vi "PH_ImageCoG_Plotter.PC Set Beam Analysis.vi"(0 "i ref in":refnum<vi>, 2 "On / Off":bool, 5 "error in (no error)":errorcluster) -> (14 "i ref out":refnum<vi>, 19 "error out":errorcluster)   [LabVIEW 2014, in "PH_ImageCoG_Plotter.lvlib"]
doc: "This VI writes beam analysis settings to own attributes and sets the GUI elements."
uses:
  PH_ImageCoG_Plotter.lvlib
  PH_Common/PH_Common.lvlib
  CSCore/BaseProcess/BaseProcess.lvlib
  PH_Img_BaseClass/PH_Img_BaseClass.lvlib
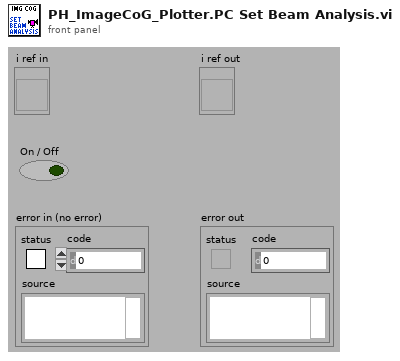
[diagram p1: front panel]
types:
  T1 = typedef "PH_ImageCoG_Plotter.lvlib/PH_ImageCoG_Plotter.i attribute.ctl" = cluster{"GUI Refs":cluster{"Delete":refnum<vi>, "Calibration status":refnum<vi>, "BI subtracted":refnum<vi>, "calc Beam Anal":refnum<vi>, "CoG - x":refnum<vi>, "CoG - y":refnum<vi>, "Type":refnum<vi>, "Center":refnum<vi>, "exp - X":refnum<vi>, "exp - Y":refnum<vi>, "Delta - X":refnum<vi>, "Delta - Y":refnum<vi>, "Available Cams":refnum<vi>, "CoG X":refnum<vi>, "CoG Y":refnum<vi>, "Delta X":refnum<vi>, "Delta Y":refnum<vi>, "Export Data":refnum<vi>, "Calibration data":refnum<vi>}, "Calibration":cluster{"Status":T2, "Calibration data":T3, "Calibration Data File":path}, "Beam Analysis":cluster{"on":bool, "exp - X":i32, "exp - Y":i32, "Type":bool, "Data":cluster{"current time":timestamp, "CoG-x":dbl, "CoG-y":dbl, "Delta-x":dbl, "Delta-y":dbl}[], "Datasets strored":i32, "Dataarray Size":i32}, "Cam instances":string[], "DIM Service Events":T4[], "Images":cluster{"Background":T7, "OP":T7, "GUI":T7}}
  T2 = typedef "PH_StatusHandler.lvlib/PH_StatusHandler.Status.ctl" = i16
  T3 = typedef "PH_ImageCalibrator.lvlib/PH_ImageCalibrator.Calibration Data.ctl" = cluster{"Date":string, "Time":string, "Cam Settings":cluster{"Cam ID":string, "Gain":dbl, "Brightness":dbl, "Shutter":dbl, "Cam Error":bool, "Mode":i32}, "Background Image":cluster{"Image":dbl[][], "Image Error":bool}, "Linear Calibration":cluster{"Calibration Factor":dbl, "not mm or mrad":bool}, "Energy Calibration":cluster{"Calibration Factor":dbl, "no mJ":bool}}
  T4 = typedef "BaseProcess.lvlib/BaseProcess.event definition.ctl" = cluster{"CAEEvtDef":T5, "Data Descriptor":T6}
  T5 = typedef "CAEObj.lvlib/CAEObj.event definition.ctl" = cluster{"URL":string, "enable":bool, "ignoreResID":bool}
  T6 = typedef "BaseProcess.lvlib/BaseProcess.descriptor string definition.ctl" = string
  T7 = typedef "IMAQ Image.ctl" = refnum<image>
  T8 = typedef "PH_Img_BaseClass.lvlib/PH_Img_BaseClass.i attribute.ctl" = cluster{"GUI Refs":T9, "Timeout Image [ms]":i32, "Default Periodic Period [ms]":i32, "Camera":cluster{"Instancename":string, "Notifier":refnum<notifier>}, "Palette":T10, "Cam Settings":cluster{"Cam ID":string, "Gain":dbl, "Brightness":dbl, "Shutter":dbl, "Cam Info Failure":bool, "Mode":i32}}
  T9 = typedef "PH_Img_BaseClass.lvlib/PH_Img_BaseClass.GUI Refs.ctl" = cluster{"Timeout":refnum<vi>, "Image":refnum<vi>, "Palette":refnum<vi>, "Timeout Set":refnum<vi>}
  T10 = typedef "PH_Img_BaseClass.lvlib/PH_Img_BaseClass.Palette.ctl" = i32
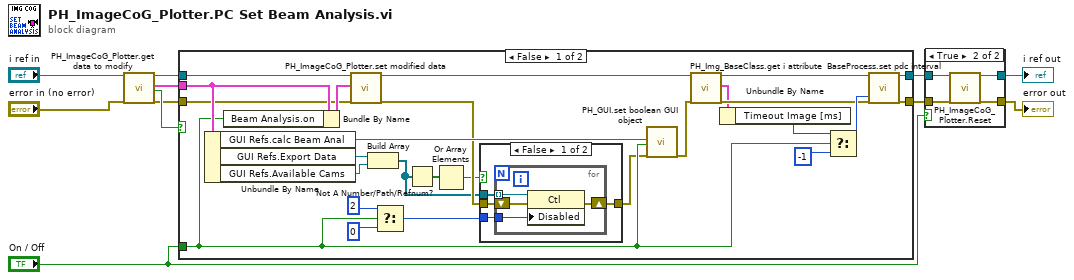
[diagram p0: block diagram]
diagram:
  n1 = call "PH_ImageCoG_Plotter.get data to modify.vi"("i ref in"="i ref in", "error in (no error)"="error in (no error)") -> ("i ref out"=w8:refnum<vi>, "i attribute"=w11:T1, "timed out"=w10:bool, "error out"=w9:errorcluster)  [unwired: 14 in]
  n2 = case shown="False" w10 {
    tunnel: w8 -> [w33 w48]
    tunnel: [w31 w48] -> w4
    tunnel: w9 -> [w28 w47]
    tunnel: [w30 w47] -> w2
    tunnel: w11 -> [w29 _]
    tunnel: "On / Off" -> [w27 _]
    frame False {
      n3 = Unbundle By Name(w29) -> ("GUI Refs.calc Beam Anal"=w34:refnum<vi>, "GUI Refs.Export Data"=w21:refnum<vi>, "GUI Refs.Available Cams"=w19:refnum<vi>)
      n4 = Bundle By Name(cluster=w29, "Beam Analysis.on"=w27) -> (w37:T1)
      n5 = call "PH_ImageCoG_Plotter.set modified data.vi"("i ref in"=w33, "i attribute"=w37, "error in (no error)"=w28) -> ("i ref out"=w32:refnum<vi>, "error out"=w26:errorcluster)  [unwired: 15 in]
      n6 = Build Array(w21, w19) -> (w20:refnum<vi>[])
      n7 = Select(t=2, s=w27, f=0) -> (s? t:f=w24:i32)
      n8 = Not A Number/Path/Refnum?(number/path/refnum=w20) -> (NaN/Path/Refnum?=w18:bool[])
      n9 = Or Array Elements(Boolean array=w18) -> (logical OR=w17:bool)
      n10 = case shown="False" w17 {
        tunnel: w26 -> [w41 w46]
        tunnel: [w40 w46] -> w25
        tunnel: w20 -> [w39 _]
        tunnel: w24 -> [w38 _]
        frame False {
          n11 = for {
            tunnel: w39 -> [w43] mode=indexing
            tunnel: w38 -> [w42]
            shift-right: [w44] -> w40
            shift-left: w41 -> [w45]
            n12 = property class="Ctl"(reference=w43, error in=w45, "Disabled"=w42) -> (error out=w44:errorcluster)  [unwired: 1 out]
          }
        }
        frame True {
        }
      }
      n13 = call "PH_GUI.set boolean GUI object.vi"("Boolean Knob GUI Ref"=w34, "Value"=w27, "error in (no error)"=w25) -> ("error out"=w15:errorcluster)  [unwired: 16 in]
      n14 = call "PH_Img_BaseClass.get i attribute.vi"("i ref in"=w32, "error in (no error)"=w15) -> ("i ref out"=w16:refnum<vi>, "i attribute"=w13:T8, "error out"=w14:errorcluster)  [unwired: 15 in]
      n15 = Unbundle By Name(w13) -> ("Timeout Image [ms]"=w12:i32)
      n16 = Select(t=w12, s=w27, f=-1 ("PeriodicInterval")) -> (s? t:f=w36:i32)
      n17 = call "BaseProcess.set pdc interval.vi"("i ref in"=w16, "PeriodicInterval [ms]"=w36, "error in (no error)"=w14) -> ("i ref out"=w31:refnum<vi>, "error out"=w30:errorcluster)  [unwired: 14 in, 1 out]
    }
    frame True {
    }
  }
  n18 = case shown="True" "On / Off" {
    tunnel: [w50 w54] -> w5
    tunnel: w4 -> [w50 w53]
    tunnel: [w49 w52] -> w3
    tunnel: w2 -> [w49 w51]
    frame False {
    }
    frame True {
      n19 = call "PH_ImageCoG_Plotter.Reset.vi"("i ref in"=w53, "error in"=w51) -> ("i ref out"=w54:refnum<vi>, "error out"=w52:errorcluster)  [unwired: 16 in]
    }
  }
  "error out" <- w3
  "i ref out" <- w5
